vi "Saturation Start Sequence.vi"(3 "error in (no error)":errorcluster, 4 "Saturation Start Angle":dbl=90.0, 5 "Rotation stage refnum":refnum<k24>) -> (0 "error out":errorcluster, 1 "Rotation stage refnum out":refnum<k24>, 2 "return position":dbl)   [LabVIEW 2023]
uses:
  C:/Users/nanometa/Documents/Thorlabs Controls/ThorLabs.MotionControl.KCube.DCServoCLI.dll
  Thorlabs Controls/ThorLabs.MotionControl.KCube.DCServoCLI.dll
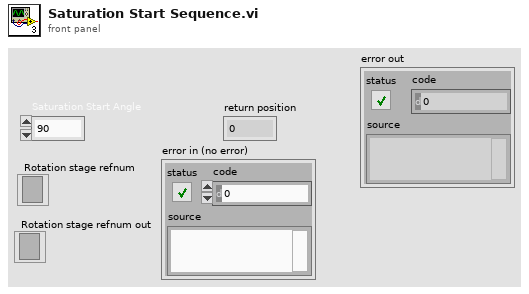
[diagram p1: front panel]
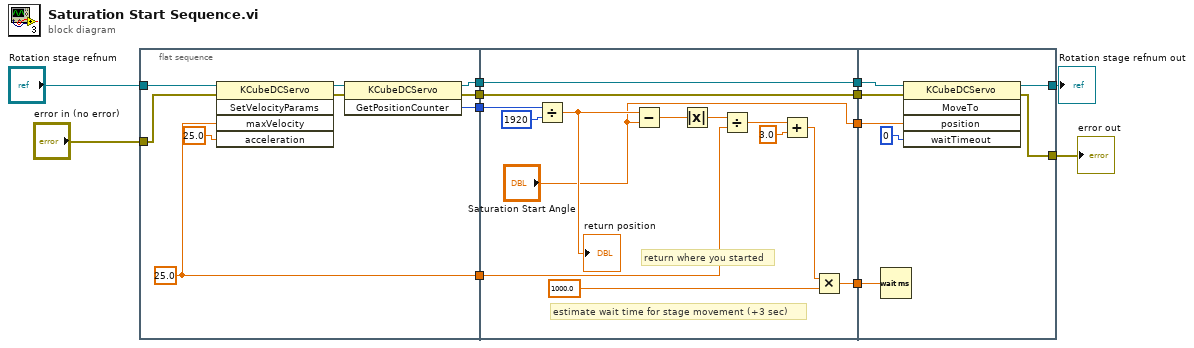
[diagram p0: block diagram]
diagram:
  n1 = flat-sequence {
    tunnel: [w20] -> w12
    tunnel: [w18] -> w11
    tunnel: [w17] -> w10
    tunnel: "Rotation stage refnum" -> [w16]
    tunnel: [w14] -> w4
    tunnel: "error in (no error)" -> [w13]
    tunnel: w12 -> [w27]
    tunnel: [w26] -> w9
    tunnel: w11 -> [w26]
    tunnel: [w25] -> w8
    tunnel: ["Saturation Start Angle"] -> w7
    tunnel: w10 -> [w23]
    tunnel: [w22] -> w5
    tunnel: w4 -> [w22]
    tunnel: w9 -> [w41]
    tunnel: w8 -> [w40]
    tunnel: w7 -> [w39]
    tunnel: w5 -> [w38]
    tunnel: [w37] -> w3
    tunnel: [w36] -> w1
    frame #0 {
      w17 = 25.0 ("maxVelocity")
      n2 = invoke class="KCubeDCServo" method="SetVelocityParams"(reference=w16, error in=w13, "maxVelocity"=w17, "acceleration"=25.0) -> (reference out=w15:refnum<k24>, error out=w19:errorcluster)  [unwired: 1 in, 3 out]
      n3 = invoke class="KCubeDCServo" method="GetPositionCounter"(reference=w15, error in=w19) -> (reference out=w14:refnum<k24>, error out=w18:errorcluster, "GetPositionCounter"=w20:i32)  [unwired: 1 in]
    }
    frame #1 {
      # "return where you started"
      # "estimate wait time for stage movement (+3 sec)"
      n4 = Divide(x=w27, y=1920) -> (x/y=w34:dbl)
      "return position" <- w34
      n5 = Subtract(x=w34, y="Saturation Start Angle") -> (x-y=w35:dbl)
      n6 = Absolute Value(x=w35) -> (abs(x)=w32:dbl)
      n7 = Divide(x=w32, y=w23) -> (x/y=w31:dbl)
      n8 = Add(x=w31, y=3.0) -> (x+y=w29:dbl)
      n9 = Multiply(x=w29, y=1000.0) -> (x*y=w25:dbl)
    }
    frame #2 {
      n10 = Wait (ms)(milliseconds to wait=w40) -> ()  [unwired: 1 out]
      n11 = invoke class="KCubeDCServo" method="MoveTo"(reference=w38, error in=w41, "position"=w39, "waitTimeout"=0) -> (reference out=w37:refnum<k24>, error out=w36:errorcluster)  [unwired: 1 in, 3 out]
    }
  }
  "Rotation stage refnum out" <- w3
  "error out" <- w1
